vi "CohortSetElectd.vi"(0 "Electd Ref":refnum<vi>, 1 "Index":u8, 2 "Amplitude":sgl) -> ()   [LabVIEW 2012, in "Cohort.lvclass"]
uses:
  Cohort.lvclass
  StimulCtrls.lvlib
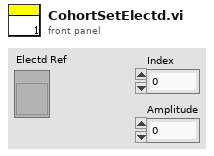
[diagram p1: front panel]
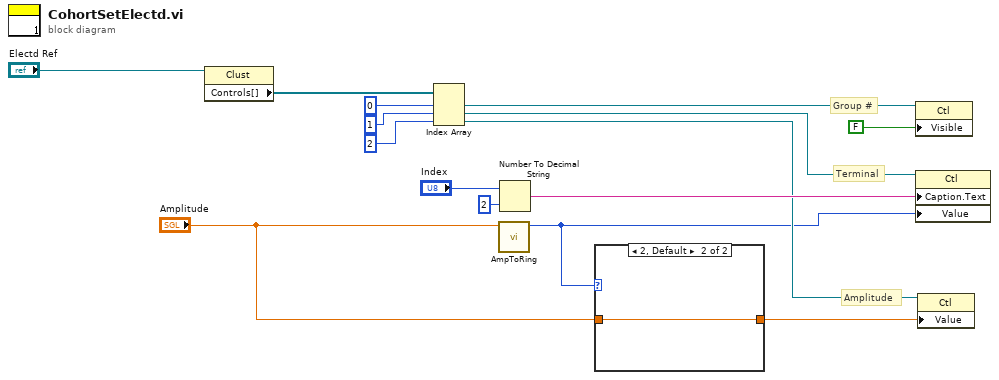
[diagram p0: block diagram]
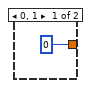
[diagram p2: hidden frame]
diagram:
  # "Amplitude"
  # "Terminal"
  # "Group #"
  n1 = property class="Clust"(reference="Electd Ref") -> ("Controls[]"=w12:refnum<vi>[])  [unwired: 1 in, 2 out]
  n2 = Index Array(array=w12, index #1=0 ("index"), index #2=1 ("index"), index #3=2 ("index")) -> (element #1=w10:refnum<vi>, element #2=w6:refnum<vi>, element #3=w4:refnum<vi>)
  n3 = call "AmpToRing.vi"("Amplitude"="Amplitude") -> ("Ring Value"=w3:u8)  [unwired: 10 in]
  n4 = Number To Decimal String(number="Index", width (-)=i16 2) -> (decimal integer string=w5:string)
  n5 = case shown="2, Default" w3 {
    tunnel: [0 w17] -> w2
    tunnel: "Amplitude" -> [_ w17]
    frame 0, 1 {
    }
    frame 2, Default {
    }
  }
  n6 = property class="Ctl"(reference=w10, "Visible"=FALSE) -> ()  [unwired: 1 in, 2 out]
  n7 = property class="Ctl"(reference=w6, "Caption.Text"=w5, "Value"=w3) -> ()  [unwired: 1 in, 2 out]
  n8 = property class="Ctl"(reference=w4, "Value"=w2) -> ()  [unwired: 1 in, 2 out]
